vi "Create Function String (Harmonics).vi"(8 "error in (no error)":errorcluster, 9 "Element/Wiring Unit (1: 1)":i32(ring)=1 items=["Null", "1", "2", "3", "4", "5", "6", "Sigma A", "Sigma B", "Sigma C"], 10 "Function (0: Uthd)":i32(ring) items=["Uthd", "Ithd", "Pthd", "Uthf", "Ithf", "Utif", "Itif", "hvf", "hcf", "K-factor", "Phi Ui-Uj", "Phi Ui-Uk", "Phi Ui-Ii", "Phi Uj-Ij", "Phi Uk-Ik"], 11 "VISA resource name":refnum<visa-resource-name>) -> (0 "error out":errorcluster, 2 "Function String":string, 3 "VISA resource name out":refnum<visa-resource-name>)   [LabVIEW 2021, in "Yokogawa WT1800 Series.lvlib"]
doc: "Create a harmonics function string.\n\n<b>Note:</b>\nThis setting valid on models with the harmonic\nmeasurement (/G5 or /G6) option."
uses:
  <instrlib>/Yokogawa WT1800 Series/Yokogawa WT1800 Series.lvlib
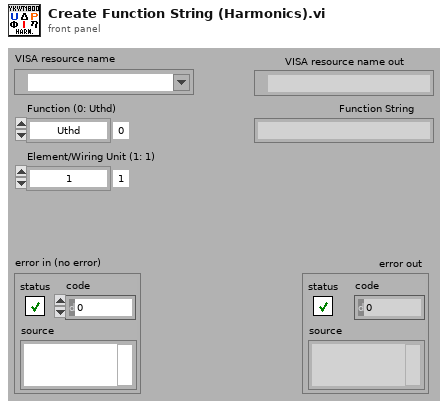
[diagram p1: front panel]
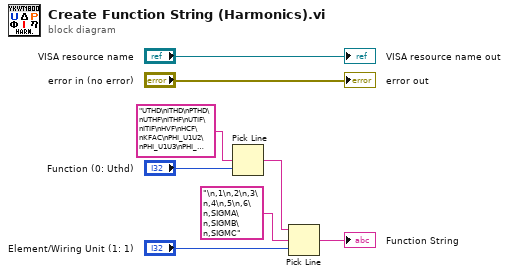
[diagram p0: block diagram]
diagram:
  n1 = Pick Line ("ライン選択")(multi-line string="UTHD\nITHD\nPTHD\nUTHF\nITHF\nUTIF\nITIF\nHVF\nHCF\nKFAC\nPHI_U1U2\nPHI_U1U3\nPHI_U1I1\nPHI_U2I2\nPHI_U3I3" ("複数行文字列"), line index="Function (0: Uthd)") -> (output string=w4:string)  [unwired: 1 in]
  n2 = Pick Line ("ライン選択")(string ("")=w4, multi-line string="\n,1\n,2\n,3\n,4\n,5\n,6\n,SIGMA\n,SIGMB\n,SIGMC" ("複数行文字列"), line index="Element/Wiring Unit (1: 1)") -> (output string=→"Function String":string)
  "VISA resource name out" <- "VISA resource name"
  "error out" <- "error in (no error)"
